vi "XYZStage-Read position command (ver 2).vi"(7 "UI ctrl refs":T1, 8 "error in (no error)":errorcluster, 11 "XYZ Stage Control.lvclass":refnum<class "XYZ Stage Control.lvclass">) -> (0 "error out":errorcluster, 2 "Coordinates":cluster{"X":sgl, "Y":sgl, "Z":sgl}, 3 "XYZ Stage Control.lvclass":refnum<class "XYZ Stage Control.lvclass">)   [LabVIEW 2020]
doc: "Reads the XYZ Stage coordinates"
uses:
  Typedefs/UI ctrl refs cluster.ctl
  Typedefs/Laser control knob.ctl
  Typedefs/Frame Size.ctl
  Typedefs/Plane Mode.ctl
  Typedefs/PMT control knob.ctl
  Typedefs/XY Stage_Move.ctl
  Typedefs/test_fpga_control.ctl
  Acquisition/Typedefs/Ref DAQ Param.ctl
  User Interface/Misc/Experiment Type.ctl
  User Interface/Misc/Biology Information.ctl
  XYZ Stage Control/XYZ Stage Control.lvclass
  <userlib>/_MGI/Application Control/MGI Change Detector/MGI Change Detector (T).vi
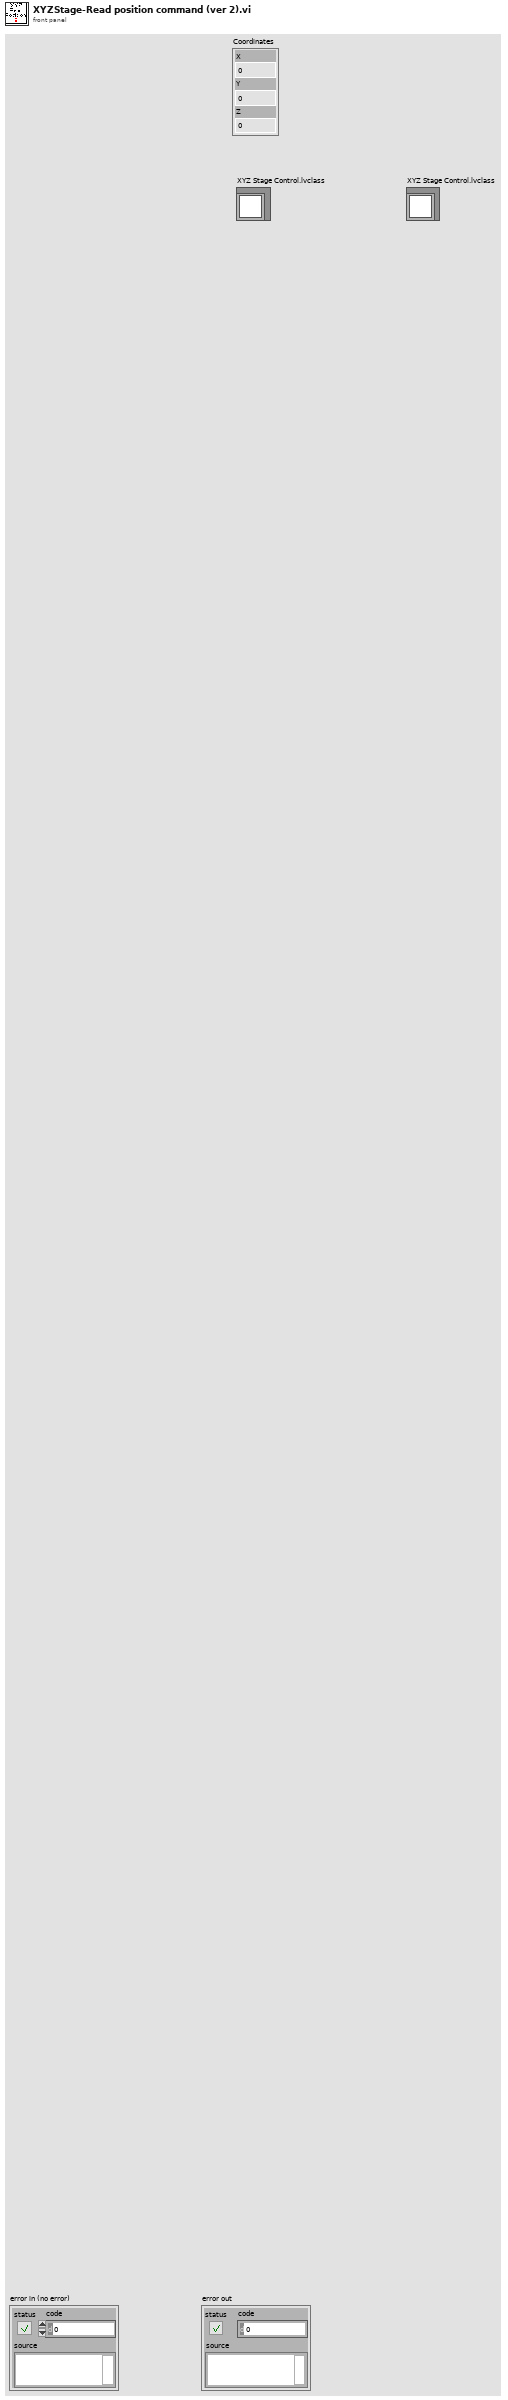
[diagram p1: front panel]
types:
  T1 = typedef "UI ctrl refs cluster.ctl" = cluster{"Top level VI path":path, "Top level VI ref":refnum<vi>, "User menu ref":refnum<k9>, "Sub Panel control":refnum<vi>, "Imaging Param Tab":refnum<vi>, "Occurrence-Start drivers":refnum<k4>, "Occurrence-Speed logging initialised":refnum<k4>, "Occurrence-XYZ stage initialised":refnum<k4>, "Exit button":refnum<vi>, "Status ind":refnum<vi>, "Set as origin":refnum<vi>, "Speed Logging":refnum<vi>, "Time Lapse":refnum<vi>, "Live Imaging":refnum<vi>, "AOL Z Stack":refnum<vi>, "Motor Z Stack":refnum<vi>, "Funct Acq button":refnum<vi>, "Hard Shutter":refnum<vi>, "Virtual Shutter":refnum<vi>, "Laser Power":refnum<vi>, "AOL Mode":refnum<vi>, "Frame Size":refnum<vi>, "Field of View":refnum<vi>, "Dwell Time":refnum<vi>, "Zoom":refnum<vi>, "AOL Z":refnum<vi>, "Objective":refnum<vi>, "Axis":refnum<vi>, "Paths & Names":refnum<vi>, "Experiment folder path (ind.)":refnum<vi>, "Last State (Ind.)":refnum<vi>, "Averages":refnum<vi>, "Angle (degrees)":refnum<vi>, "X centre":refnum<vi>, "Y centre":refnum<vi>, "Plane Mode":refnum<vi>, "# Planes":refnum<vi>, "Z Start":refnum<vi>, "Z Stop":refnum<vi>, "Z Step":refnum<vi>, "PMT 1":refnum<vi>, "PMT 2":refnum<vi>, "Stage XYZ Position":refnum<vi>, "Pockels@Z Start":refnum<vi>, "Pockels@Z Stop":refnum<vi>, "Obtain Z Start":refnum<vi>, "Obtain Z Stop":refnum<vi>, "Live stim.trig.period":refnum<vi>, "Live stim.trig.enable":refnum<vi>, "Movement Correction":refnum<vi>, "Load Reference Image":refnum<vi>, "XY Stage Move":refnum<vi>, "MovCor Cluster":refnum<vi>, "RefDAQParam":refnum<vi>, "Funct. Acq. Pockels Modulation":refnum<vi>, "Ref Laser Power":refnum<vi>, "Enable Video Recording":refnum<vi>, "Video Record-Live Imaging":refnum<vi>, "Video Record-Funct acq":refnum<vi>, "Reference Source":refnum<vi>, "AOL Z-stack Chirps Ready (ind)":refnum<vi>, "Target time between mov.cor. ref triggers (ms)":refnum<vi>, "Funct. Acq. Ref frame save":refnum<vi>, "Tracking button":refnum<vi>, "Show ref plots window":refnum<vi>, "Center freq ind (nm)":refnum<vi>, "Pickup mode (ind)":refnum<vi>, "Logging queue (ind)":refnum<vi>, "Back aperture power (ind.)":refnum<vi>, "Power after objective (ind.)":refnum<vi>, "Switch user":refnum<vi>, "Ls1 Conn. Status":refnum<vi>, "Ls1Tuning Status":refnum<vi>, "Ls1 Faults":refnum<vi>, "Ls1 Connection":refnum<vi>, "Ls1 Mode":refnum<vi>, "Ls1 POWER [mW]":refnum<vi>, "Ls1Shutter":refnum<vi>, "Ls1 Wavelength":refnum<vi>, "Ls1 Note":refnum<vi>, "Ls1 Confirm Wav":refnum<vi>, "Ls1 PreChrp Prism1":refnum<vi>, "Ls1 PreChrp Prism2":refnum<vi>, "Ls1 wav top Ind":refnum<vi>, "Ls1 power top Ind":refnum<vi>, "Ls1 Pump peak Hold":refnum<vi>, "Ls1 Status Ind":refnum<vi>, "Ls1 wav cancel":refnum<vi>, "Experiment Type":refnum<vi>, "Biology Information":refnum<vi>, "Camera recording status":refnum<vi>, "Optimise Obj. Pos.":refnum<vi>}
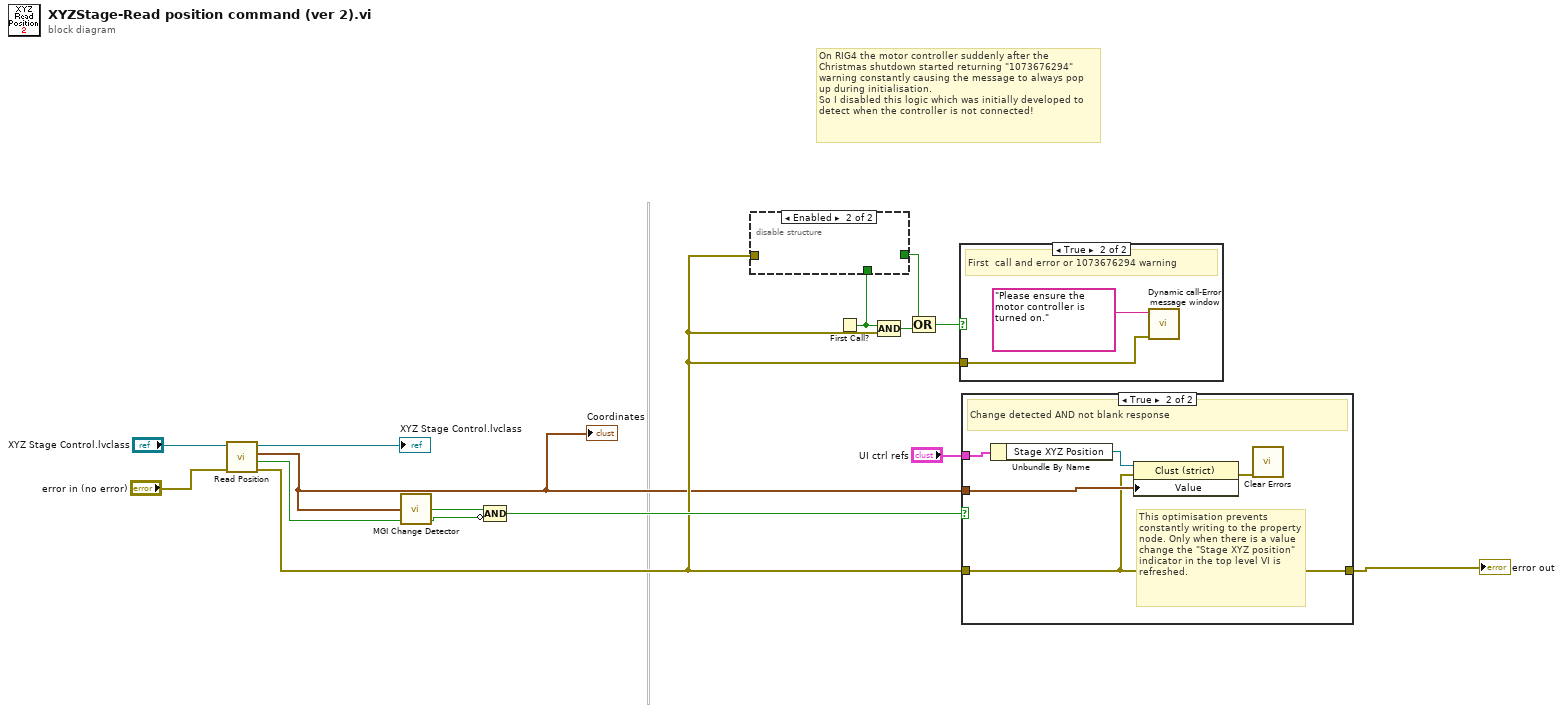
[diagram p0: block diagram]
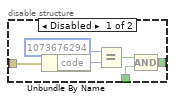
[diagram p2: hidden frame]
diagram:
  # "On RIG4 the motor controller suddenly after the Christmas shutdown started returning \"1073676294\" warning constantly causing the message to always pop up during initialisation.\nSo I disabled this logic which was initially developed to detect when the controller is not connected!"
  n1 = call-dynamic "Read Position.vi"("error in (no error)"="error in (no error)", "XYZ Stage Control in"="XYZ Stage Control.lvclass") -> ("error out"=w7:errorcluster, "No Feedback"=w1:bool, "Stage XYZ Position"=w5:cluster{"X":sgl, "Y":sgl, "Z":sgl}, "XYZ Stage Control out"=→"XYZ Stage Control.lvclass":refnum<class "XYZ Stage Control.lvclass">)  [unwired: 6 in]
  "Coordinates" <- w5
  n2 = call-poly <userlib>:"MGI Change Detector.vi"("Value"=w5) -> ("Changed?"=w2:bool)
  n3 = Compound Arithmetic op=AND(w2, invert w1) -> (w12:bool)
  n4 = First Call?() -> (First Call?: T/F=w10:bool)
  n5 = disable-structure shown="Enabled" {
    disable-tunnel: [w17 _] -> w11
    disable-tunnel: w10 -> [w16 _]
    disable-tunnel: w7 -> [w15 _]
    frame Disabled {
      n6 = Unbundle By Name(w15) -> ("code"=w20:i32)
      n7 = Equal?(x=1073676294, y=w20) -> (x = y?=w18:bool)
      n8 = Compound Arithmetic op=AND(w18, w16) -> (w17:bool)
    }
    frame Enabled {
    }
  }
  n9 = Compound Arithmetic op=AND(w10, w7) -> (w9:bool)
  n10 = Compound Arithmetic op=OR(w11, w9) -> (w8:bool)
  n11 = case shown="True" w8 {
    tunnel: w7 -> [_ w21]
    frame False {
    }
    frame True {
      # "First  call and error or 1073676294 warning"
      n12 = call "Dynamic call-Error message window.vi"("error in (no error)"=w21, "Error Message"="Please ensure the motor controller is turned on.") -> ()  [unwired: 9 in, 1 out]
    }
  }
  n13 = case shown="True" w12 {
    tunnel: [w23 w24] -> w14
    tunnel: w7 -> [w23 w24]
    tunnel: w5 -> [_ w28]
    tunnel: "UI ctrl refs" -> [_ w27]
    frame False {
      # "No change OR blank response"
    }
    frame True {
      # "This optimisation prevents constantly writing to the property node. Only when there is a value change the \"Stage XYZ position\" indicator in the top level VI is refreshed."
      # "Change detected AND not blank response"
      n14 = Unbundle By Name(w27) -> ("Stage XYZ Position"=w26:refnum<vi>)
      n15 = property on="Property Node" class="Clust (strict)"(reference=w26, error in=w24, "Value"=w28) -> (error out=w25:errorcluster)  [unwired: 1 out]
      n16 = call <vilib>:"Clear Errors.vi"("error in (no error)"=w25) -> ()  [unwired: 5 in, 2 out]
    }
  }
  "error out" <- w14
